vi "FPGA_EncoderReadTimerOutput.vi"(8 "error in (no error)":errorcluster, 11 "EncoderDevRef":T1) -> (0 "error out":errorcluster, 1 "Stalled":bool, 2 "Period (s)":dbl, 3 "EncoderDevRef":T1)   [LabVIEW 2017]
uses:
  <vilib>/Rock Robotics/SystemInterfaces/Encoder/FPGA_EncoderDevRef.ctl
  <vilib>/Rock Robotics/SystemInterfaces/Encoder/FPGA_EncoderIdx.ctl
  <vilib>/Rock Robotics/SystemInterfaces/System/FPGA_SystemFPGA Ref Global.vi
  <vilib>/Utility/error.llb/Error Cluster From Error Code.vi
  <vilib>/rvi/errors/niLvFpgaAdjustHostInterfaceError.vi
  <vilib>/rvi/interface/nirviReadWriteControl/nirviReadWriteControl.xnode
  <vilib>/Rock Robotics/SystemInterfaces/System/FPGA_SystemFRC FPGA Ref.ctl
  NiFpgaLv.dll
  <vilib>/rvi/interface/Simulation/niFpgaSimulationCallBeginRW.vi
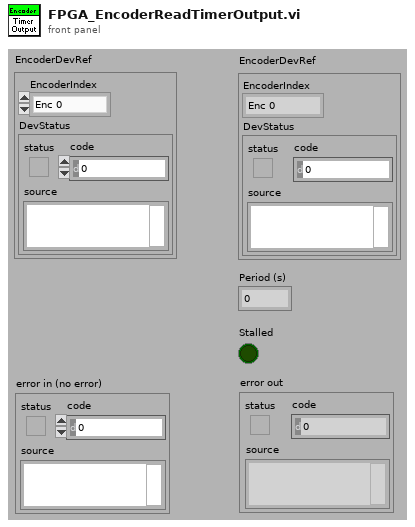
[diagram p1: front panel]
types:
  T1 = typedef "FPGA_EncoderDevRef.ctl" = cluster{"EncoderIndex":T2, "DevStatus":errorcluster}
  T2 = typedef "FPGA_EncoderIdx.ctl" = enum8{"Enc 0", "Enc 1", "Enc 2", "Enc 3", "Enc 4", "Enc 5", "Enc 6", "Enc 7", "Invalid"}
  T3 = typedef "FPGA_SystemFRC FPGA Ref.ctl" = refnum<k20>
  T4 = cluster{"Period":fxp<+,23,24>, "Count":fxp<+/-,8,8>, "Stalled":bool}
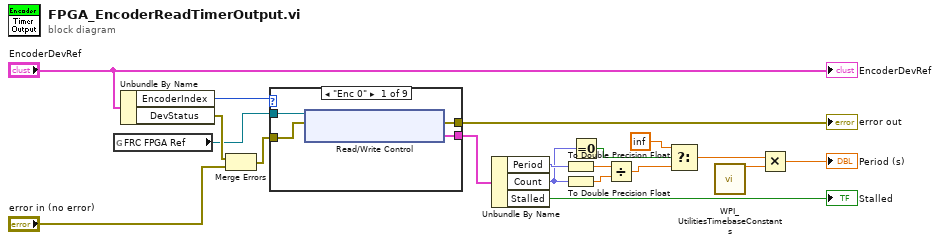
[diagram p0: block diagram]
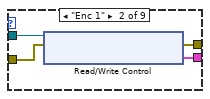
[diagram p2: hidden frame]
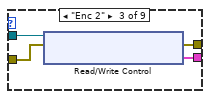
[diagram p3: hidden frame]
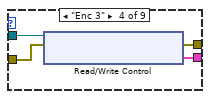
[diagram p4: hidden frame]
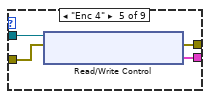
[diagram p5: hidden frame]
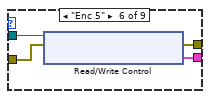
[diagram p6: hidden frame]
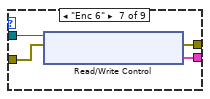
[diagram p7: hidden frame]
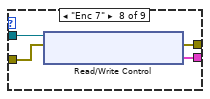
[diagram p8: hidden frame]
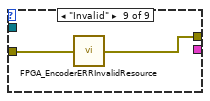
[diagram p9: hidden frame]
diagram:
  n1 = global read "FPGA_SystemFPGA Ref Global.vi" "FRC FPGA Ref"() -> (w3:T3)
  n2 = Unbundle By Name("EncoderDevRef") -> ("EncoderIndex"=w15:T2, "DevStatus"=w5:errorcluster)
  n3 = Merge Errors(w5, "error in (no error)") -> (w4:errorcluster)
  n4 = case shown="\"Enc 0\"" w15 {
    tunnel: w3 -> [w21 w25 w29 w33 w37 w41 w45 w49 _]
    tunnel: w4 -> [w22 w26 w30 w34 w38 w42 w46 w50 w53]
    tunnel: [w23 w27 w31 w35 w39 w43 w47 w51 w52] -> w18
    tunnel: [w20 w24 w28 w32 w36 w40 w44 w48 _] -> w14
    frame "Enc 0" {
      n5 = xnode "Read/Write Control"("FPGA VI Reference In"=w21, "error in"=w22) -> ("error out"=w23:errorcluster, "Encoder0.TimerOutput"=w20:T4)  [unwired: 1 out]
    }
    frame "Enc 1" {
      n6 = xnode "Read/Write Control"("FPGA VI Reference In"=w25, "error in"=w26) -> ("error out"=w27:errorcluster, "Encoder1.TimerOutput"=w24:T4)  [unwired: 1 out]
    }
    frame "Enc 2" {
      n7 = xnode "Read/Write Control"("FPGA VI Reference In"=w29, "error in"=w30) -> ("error out"=w31:errorcluster, "Encoder2.TimerOutput"=w28:T4)  [unwired: 1 out]
    }
    frame "Enc 3" {
      n8 = xnode "Read/Write Control"("FPGA VI Reference In"=w33, "error in"=w34) -> ("error out"=w35:errorcluster, "Encoder3.TimerOutput"=w32:T4)  [unwired: 1 out]
    }
    frame "Enc 4" {
      n9 = xnode "Read/Write Control"("FPGA VI Reference In"=w37, "error in"=w38) -> ("error out"=w39:errorcluster, "Encoder4.TimerOutput"=w36:T4)  [unwired: 1 out]
    }
    frame "Enc 5" {
      n10 = xnode "Read/Write Control"("FPGA VI Reference In"=w41, "error in"=w42) -> ("error out"=w43:errorcluster, "Encoder5.TimerOutput"=w40:T4)  [unwired: 1 out]
    }
    frame "Enc 6" {
      n11 = xnode "Read/Write Control"("FPGA VI Reference In"=w45, "error in"=w46) -> ("error out"=w47:errorcluster, "Encoder6.TimerOutput"=w44:T4)  [unwired: 1 out]
    }
    frame "Enc 7" {
      n12 = xnode "Read/Write Control"("FPGA VI Reference In"=w49, "error in"=w50) -> ("error out"=w51:errorcluster, "Encoder7.TimerOutput"=w48:T4)  [unwired: 1 out]
    }
    frame "Invalid" {
      n13 = call <vilib>:"FPGA_EncoderERRInvalidResource.vi"("error in (no error)"=w53) -> ("error out"=w52:errorcluster)
    }
  }
  "error out" <- w18
  n14 = Unbundle By Name(w14) -> ("Period"=w11:fxp<+,23,24>, "Count"=w9:fxp<+/-,8,8>, "Stalled"=→"Stalled":bool)
  n15 = To Double Precision Float(number=w11) -> (double precision float=w10:dbl)
  n16 = To Double Precision Float(number=w9) -> (double precision float=w8:dbl)
  n17 = Equal To 0?(x=w9) -> (x = 0?=w13:bool)
  n18 = Divide(x=w10, y=w8) -> (x/y=w6:dbl)
  n19 = Select(t=inf ("Period"), s=w13, f=w6) -> (s? t:f=w7:dbl)
  n20 = call <vilib>:"WPI_UtilitiesTimebaseConstants.vi"() -> ("40 MHz FPGA clock"=w2:dbl)  [unwired: 13 in, 2 out]
  n21 = Multiply(x=w7, y=w2) -> (x*y=→"Period (s)":dbl)
  "EncoderDevRef" <- "EncoderDevRef"
